vi "MAIN CARICA STRINGHE.vi"() -> ()   [LabVIEW 2016]
uses:
  <vilib>/Utility/file.llb/Read Delimited Spreadsheet (string).vi
panel:
  out "Array":string[](array[string])
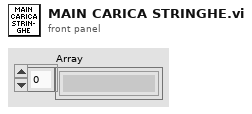
[diagram p1: front panel]
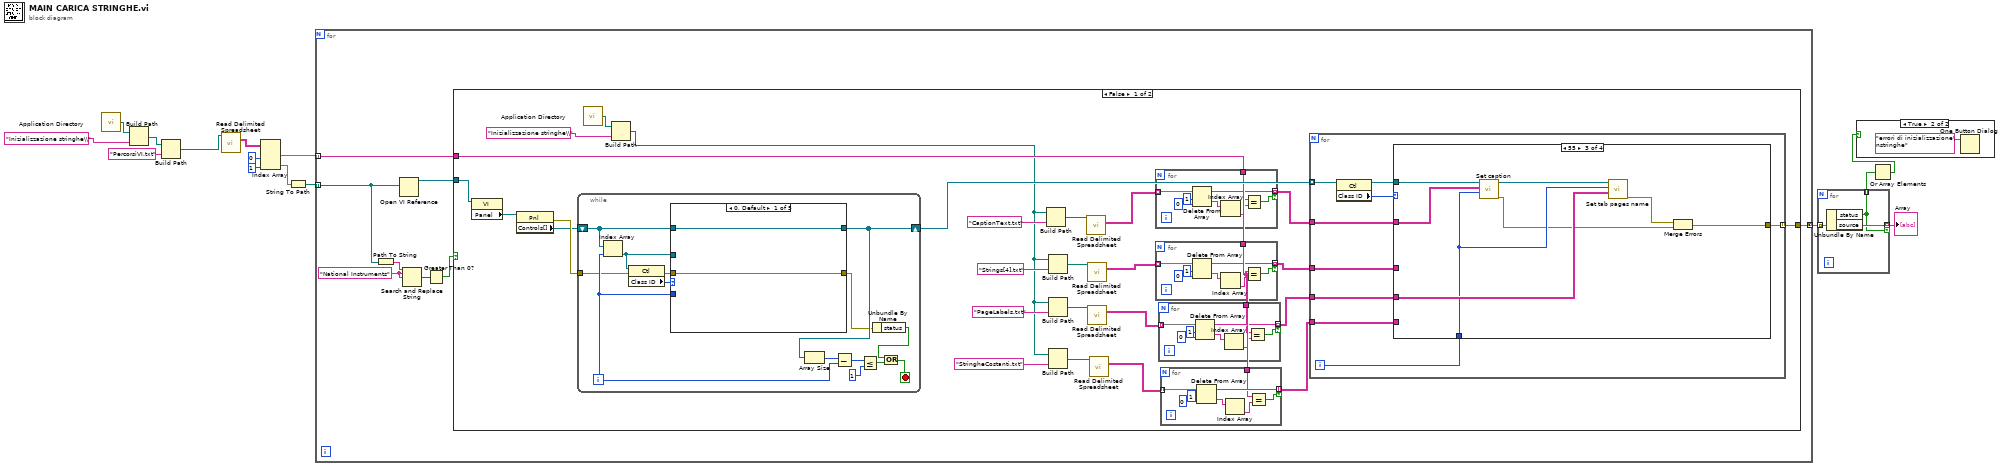
[diagram p0: block diagram]
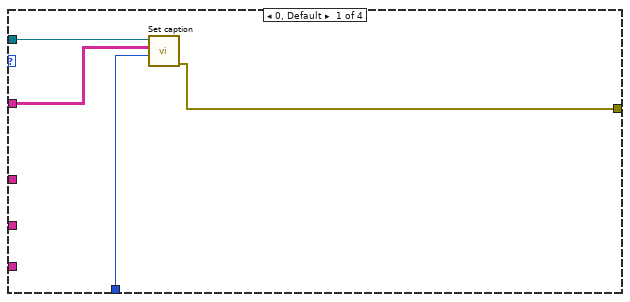
[diagram p3: hidden frame]
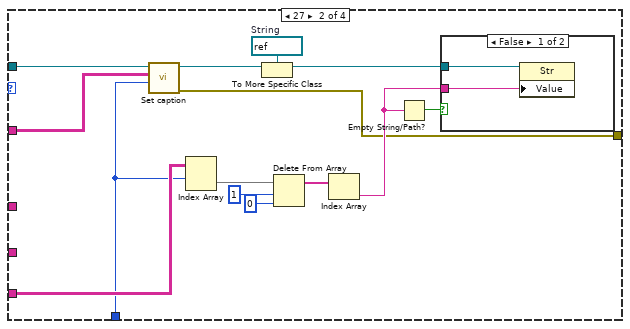
[diagram p4: hidden frame]
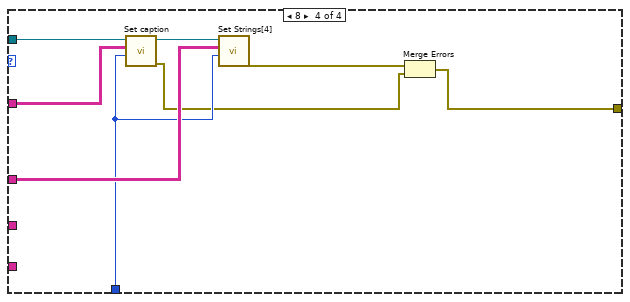
[diagram p6: hidden frame]
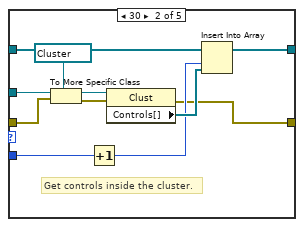
[diagram p7: hidden frame]
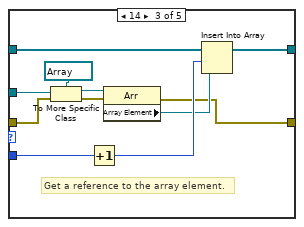
[diagram p8: hidden frame]
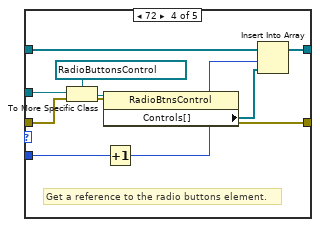
[diagram p9: hidden frame]
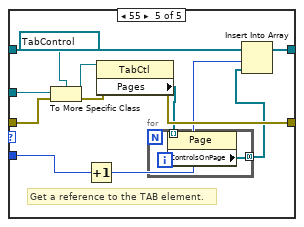
[diagram p10: hidden frame]
diagram:
  n1 = call <vilib>:"Application Directory.vi"() -> ("Application Directory"=w4:path)
  n2 = Build Path(base path=w4, name or relative path="Inizializzazione stringhe\\") -> (appended path=w5:path)
  n3 = Build Path(base path=w5, name or relative path="PercorsiVI.txt") -> (appended path=w6:path)
  n4 = call-poly <vilib>:"Read Delimited Spreadsheet.vi"("file path (dialog if empty)"=w6) -> ("all rows"=w7:string[][])  [unwired: 9 in, 5 out]
  n5 = Index Array(array=w7, index (col) #1=0 ("disabled index (col)"), index (col) #2=1 ("index (col)")) -> (element #1=w10:string[], element #2=w11:string[])  [unwired: 2 in]
  n6 = String To Path(string=w11) -> (path=w12:path[])
  n7 = for {
    tunnel: w12 -> [w21] mode=indexing
    tunnel: w10 -> [w22] mode=indexing
    tunnel: [w16] -> w15 mode=concatenating
    w19 = "National Instruments" ("search string")
    n8 = Path To String(path=w21) -> (string=w20:string)
    n9 = Open VI Reference(vi path=w21) -> (vi reference=w23:refnum<vi>)  [unwired: 5 in, 1 out]
    n10 = Search and Replace String(input string=w20, search string=w19, replace string=w19) -> (number of replacements=w18:i32)  [unwired: 5 in, 3 out]
    n11 = Greater Than 0?(x=w18) -> (x > 0?=w17:bool)
    n12 = case shown="False" w17 {
      tunnel: w23 -> [w46 _]
      tunnel: w22 -> [w31 _]
      tunnel: [w24 _] -> w16
      frame False {
        n13 = property class="VI"(reference=w46) -> ("Panel"=w47:refnum<vi>)  [unwired: 1 in, 2 out]
        n14 = property class="Pnl"(reference=w47) -> (error out=w49:errorcluster, "Controls[]"=w48:refnum<vi>[])  [unwired: 1 in, 1 out]
        n15 = while {
          shift-right: [w131] -> w37
          shift-left: w48 -> [w132]
          tunnel: w49 -> [w130]
          i -> [w137]
          stop <- w135 stop-if-true
          n16 = Index Array(array=w132, index=w137) -> (element=w133:refnum<vi>)
          n17 = property class="Ctl"(reference=w133, error in=w130) -> (error out=w129:errorcluster, "Class ID"=w134:u32)  [unwired: 1 out]
          n18 = case shown="0, Default" w134 {
            tunnel: w133 -> [_ w153 w164 w175 w187]
            tunnel: w132 -> [w142 w150 w161 w174 w186]
            tunnel: w137 -> [_ w149 w160 w173 w185]
            tunnel: [w142 w147 w159 w172 w184] -> w131
            tunnel: w129 -> [w141 w145 w156 w171 w183]
            tunnel: [w141 w143 w154 w170 w182] -> w127
            frame 0, Default {
            }
            frame 30 {
              # "Get controls inside the cluster."
              n19 = To More Specific Class(target class=refnum<vi> refnum ("target class 3"), reference=w153, error in=w145) -> (specific class reference=w152:refnum<vi>, error out=w144:errorcluster)
              n20 = Increment(x=w149) -> (x+1=w146:i32)
              n21 = property class="Clust"(reference=w152, error in=w144) -> (error out=w143:errorcluster, "Controls[]"=w148:refnum<vi>[])  [unwired: 1 out]
              n22 = Insert Into Array(array=w150, index=w146, new element=w148) -> (w147:refnum<vi>[])
            }
            frame 14 {
              # "Get a reference to the array element."
              n23 = To More Specific Class(target class=refnum<vi> refnum ("target class 4"), reference=w164, error in=w156) -> (specific class reference=w163:refnum<vi>, error out=w155:errorcluster)
              n24 = Increment(x=w160) -> (x+1=w158:i32)
              n25 = property class="Arr"(reference=w163, error in=w155) -> (error out=w154:errorcluster, "Array Element"=w157:refnum<vi>)  [unwired: 1 out]
              n26 = Insert Into Array(array=w161, index=w158, new element=w157) -> (w159:refnum<vi>[])
            }
            frame 72 {
              # "Get a reference to the radio buttons element."
              n27 = To More Specific Class(target class=refnum<vi> refnum ("Calcolo P2"), reference=w175, error in=w171) -> (specific class reference=w169:refnum<vi>, error out=w166:errorcluster)
              n28 = property class="RadioBtnsControl"(reference=w169, error in=w166) -> (error out=w170:errorcluster, "Controls[]"=w167:refnum<vi>[])  [unwired: 1 out]
              n29 = Increment(x=w173) -> (x+1=w168:i32)
              n30 = Insert Into Array(array=w174, index=w168, new element=w167) -> (w172:refnum<vi>[])
            }
            frame 55 {
              # "Get a reference to the TAB element."
              n31 = To More Specific Class(target class=refnum<vi> refnum ("Tab Control"), reference=w187, error in=w183) -> (specific class reference=w181:refnum<vi>, error out=w179:errorcluster)
              n32 = Increment(x=w185) -> (x+1=w180:i32)
              n33 = property class="TabCtl"(reference=w181, error in=w179) -> (error out=w182:errorcluster, "Pages"=w177:refnum<vi>[])  [unwired: 1 out]
              n34 = for {
                tunnel: w177 -> [w189] mode=indexing
                tunnel: [w188] -> w176 mode=concatenating
                n35 = property class="Page"(reference=w189) -> ("ControlsOnPage"=w188:refnum<vi>[])  [unwired: 1 in, 2 out]
              }
              n36 = Insert Into Array(array=w186, index=w180, new element=w176) -> (w184:refnum<vi>[])
            }
          }
          n37 = Array Size(array=w131) -> (size(s)=w140:i32)
          n38 = Subtract(x=w140, y=w137) -> (x-y=w139:i32)
          n39 = Less Or Equal?(x=w139, y=1) -> (x <= y?=w136:bool)
          n40 = Unbundle By Name(w127) -> ("status"=w128:bool)
          n41 = Or(x=w128, y=w136) -> (x .or. y?=w135:bool)
        }
        n42 = call <vilib>:"Application Directory.vi"() -> ("Application Directory"=w26:path)
        n43 = Build Path(base path=w26, name or relative path="Inizializzazione stringhe\\") -> (appended path=w25:path)
        n44 = Build Path(base path=w25, name or relative path="CaptionText.txt") -> (appended path=w45:path)
        n45 = Build Path(base path=w25, name or relative path="Strings[4].txt") -> (appended path=w40:path)
        n46 = Build Path(base path=w25, name or relative path="PageLabels.txt") -> (appended path=w39:path)
        n47 = Build Path(base path=w25, name or relative path="StringheCostanti.txt") -> (appended path=w38:path)
        n48 = call-poly <vilib>:"Read Delimited Spreadsheet.vi"("file path (dialog if empty)"=w45) -> ("all rows"=w36:string[][])  [unwired: 9 in, 5 out]
        n49 = call-poly <vilib>:"Read Delimited Spreadsheet.vi"("file path (dialog if empty)"=w40) -> ("all rows"=w34:string[][])  [unwired: 9 in, 5 out]
        n50 = call-poly <vilib>:"Read Delimited Spreadsheet.vi"("file path (dialog if empty)"=w39) -> ("all rows"=w33:string[][])  [unwired: 9 in, 5 out]
        n51 = call-poly <vilib>:"Read Delimited Spreadsheet.vi"("file path (dialog if empty)"=w38) -> ("all rows"=w32:string[][])  [unwired: 9 in, 5 out]
        n52 = for {
          tunnel: w36 -> [w81] mode=indexing
          tunnel: [w77] -> w35 mode=indexing if=w75
          tunnel: w31 -> [w74]
          n53 = Delete From Array(array=w81, length=1, index=0) -> (deleted portion=w78:string[], array with subset deleted=w77:string[])
          n54 = Index Array(array=w78) -> (element=w76:string)  [unwired: 1 in]
          n55 = Equal?(x=w74, y=w76) -> (x = y?=w75:bool)
        }
        n56 = for {
          tunnel: w34 -> [w73] mode=indexing
          tunnel: [w69] -> w30 mode=indexing if=w67
          tunnel: w31 -> [w66]
          n57 = Delete From Array(array=w73, length=1, index=0) -> (deleted portion=w70:string[], array with subset deleted=w69:string[])
          n58 = Index Array(array=w70) -> (element=w68:string)  [unwired: 1 in]
          n59 = Equal?(x=w66, y=w68) -> (x = y?=w67:bool)
        }
        n60 = for {
          tunnel: w33 -> [w65] mode=indexing
          tunnel: [w61] -> w29 mode=indexing if=w59
          tunnel: w31 -> [w58]
          n61 = Delete From Array(array=w65, length=1, index=0) -> (deleted portion=w62:string[], array with subset deleted=w61:string[])
          n62 = Index Array(array=w62) -> (element=w60:string)  [unwired: 1 in]
          n63 = Equal?(x=w58, y=w60) -> (x = y?=w59:bool)
        }
        n64 = for {
          tunnel: w32 -> [w57] mode=indexing
          tunnel: [w53] -> w28 mode=indexing if=w51
          tunnel: w31 -> [w50]
          n65 = Delete From Array(array=w57, length=1, index=0) -> (deleted portion=w54:string[], array with subset deleted=w53:string[])
          n66 = Index Array(array=w54) -> (element=w52:string)  [unwired: 1 in]
          n67 = Equal?(x=w50, y=w52) -> (x = y?=w51:bool)
        }
        n68 = for {
          tunnel: w35 -> [w87]
          tunnel: w30 -> [w86]
          tunnel: w37 -> [w90] mode=indexing
          tunnel: w29 -> [w84]
          tunnel: w28 -> [w83]
          tunnel: [w82] -> w24 mode=indexing
          i -> [w85]
          n69 = property class="Ctl"(reference=w90) -> (reference out=w88:refnum<vi>, "Class ID"=w89:u32)  [unwired: 1 in, 1 out]
          n70 = case shown="55" w89 {
            tunnel: w88 -> [w94 w108 w118 w125]
            tunnel: w87 -> [w93 w107 w117 w123]
            tunnel: w86 -> [_ _ _ w126]
            tunnel: w85 -> [w92 w103 w114 w122]
            tunnel: w84 -> [_ _ w115 _]
            tunnel: w83 -> [_ w104 _ _]
            tunnel: [w91 w95 w111 w119] -> w82
            frame 0, Default {
              n71 = call "Set caption.vi"("index (row)"=w92, "Array"=w93, "Control in"=w94) -> ("error out"=w91:errorcluster)  [unwired: 7 in, 1 out]
            }
            frame 27 {
              w106 = refnum<vi> refnum  # String
              n72 = call "Set caption.vi"("index (row)"=w103, "Array"=w107, "Control in"=w108) -> ("error out"=w95:errorcluster, "reference out"=w105:refnum<vi>)  [unwired: 7 in]
              n73 = Index Array(array=w104, index (row)=w103) -> (element=w102:string[])  [unwired: 1 in]
              n74 = To More Specific Class(target class=w106, reference=w105) -> (specific class reference=w99:refnum<vi>)  [unwired: 1 in, 1 out]
              n75 = Delete From Array(array=w102, length=1, index=0) -> (array with subset deleted=w98:string[])  [unwired: 1 out]
              n76 = Index Array(array=w98) -> (element=w96:string)  [unwired: 1 in]
              n77 = Empty String/Path?(string/path=w96) -> (empty?=w97:bool)
              n78 = case shown="False" w97 {
                tunnel: w99 -> [w110 _]
                tunnel: w96 -> [w109 _]
                frame False {
                  n79 = property class="Str"(reference=w110, "Value"=w109) -> ()  [unwired: 1 in, 2 out]
                }
                frame True {
                }
              }
            }
            frame 55 {
              n80 = call "Set caption.vi"("index (row)"=w114, "Array"=w117, "Control in"=w118) -> ("error out"=w112:errorcluster, "reference out"=w116:refnum<vi>)  [unwired: 7 in]
              n81 = call "Set tab pages name.vi"("Array"=w115, "Numeric"=w114, "Control in"=w116) -> ("error out"=w113:errorcluster)  [unwired: 7 in, 1 out]
              n82 = Merge Errors(w113, w112) -> (w111:errorcluster)
            }
            frame 8 {
              n83 = call "Set caption.vi"("index (row)"=w122, "Array"=w123, "Control in"=w125) -> ("error out"=w120:errorcluster, "reference out"=w124:refnum<vi>)  [unwired: 7 in]
              n84 = call "Set Strings[4].vi"("index (row)"=w122, "Array"=w126, "Control in"=w124) -> ("error out"=w121:errorcluster)  [unwired: 7 in, 1 out]
              n85 = Merge Errors(w121, w120) -> (w119:errorcluster)
            }
          }
        }
      }
      frame True {
        # "scarta i vi nella cartella national instruments (quelli della libreria labview)"
      }
    }
  }
  n86 = for {
    tunnel: w15 -> [w192] mode=indexing
    tunnel: [w191] -> w1 mode=indexing if=w190
    tunnel: [w190] -> w14 mode=indexing
    n87 = Unbundle By Name(w192) -> ("status"=w190:bool, "source"=w191:string)
  }
  "Array" <- w1
  n88 = Or Array Elements(Boolean array=w14) -> (logical OR=w13:bool)
  n89 = case shown="True" w13 {
    frame False {
    }
    frame True {
      n90 = One Button Dialog(message="errori di inizializzazione\nstringhe") -> ()  [unwired: 1 in, 1 out]
    }
  }
